vi "Parse.vi"(8 "error in (no error)":errorcluster, 10 "Transfer Group in":refnum<class "Transfer Group.lvclass">, 11 "Type Converter in":refnum<class "Default Buffer Converter.lvclass">) -> (0 "error out":errorcluster, 2 "Transfer Group out":refnum<class "Transfer Group.lvclass">, 3 "Type Converter out":refnum<class "Default Buffer Converter.lvclass">)   [LabVIEW 2019, in "DSF Core.lvlib" / "Default Buffer Converter.lvclass"]
uses:
  Default Buffer Converter.lvclass
  Classes/Transfer Group/Transfer Group.lvclass
  Classes/Transfer Group/Transfer Group.lvclass/Transfer Group.ctl
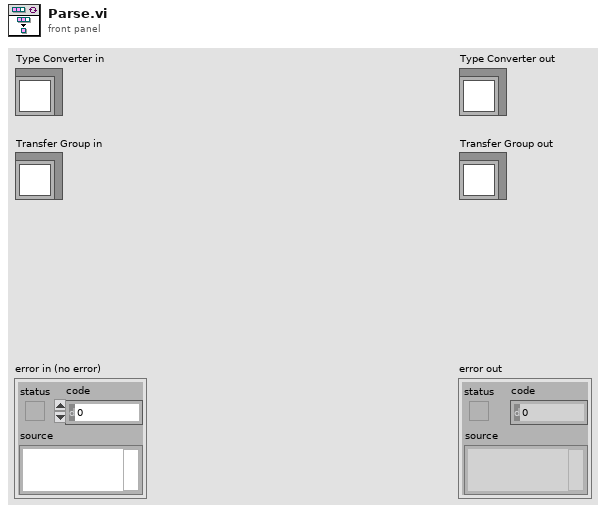
[diagram p1: front panel]
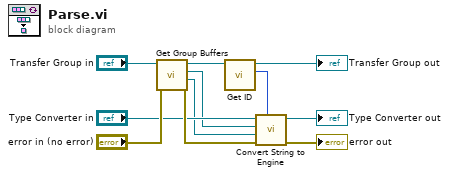
[diagram p0: block diagram]
diagram:
  n1 = call "Get Group Buffers.vi"("error in (no error)"="error in (no error)", "Transfer Group in"="Transfer Group in") -> ("error out"=w10:errorcluster, "string Buffer"=w1:refnum<class "Buffer.lvclass">, "engine Buffer"=w2:refnum<class "Buffer.lvclass">, "Transfer Group out"=w11:refnum<class "Transfer Group.lvclass">)  [unwired: 6 in]
  n2 = call "Get ID.vi"("Transfer Group in"=w11) -> ("id"=w9:i32, "Transfer Group out"=→"Transfer Group out":refnum<class "Transfer Group.lvclass">)  [unwired: 9 in]
  n3 = call-dynamic "Convert String to Engine.vi"("transfer group id"=w9, "error in"=w10, "string buffer"=w1, "engine buffer"=w2, "DSF buffer converter in"="Type Converter in") -> ("error out"=→"error out":errorcluster, "DSF buffer converter out"=→"Type Converter out":refnum<class "Default Buffer Converter.lvclass">)  [unwired: 5 in]
